vi "Memory.Pointer.Read.Safe.0D.I8.vi"(8 "error in (no error)":errorcluster, 10 "value in":i8, 11 "pointer in":refnum<class "Memory.Pointer.lvclass">) -> (0 "error out":errorcluster, 2 "value out":i8, 3 "pointer out":refnum<class "Memory.Pointer.lvclass">)   [LabVIEW 2016, in "Memory Manager.lvlib" / "Memory.Pointer.lvclass"]
doc: "Reads from the address specified by <b>pointer</b> into <b>value</b>.\n\n<b>Note:</b> This VI is <b>unsafe</b>.\n\nUnsafe means that it does not evaluate the size parameter of <b>pointer</b> to ensure that is inbounds of allocated memory before peforming a memory read/write. Reading/writing more data to a pointer than it has allocated can corrupt or crash LabVIEW. Only use this VI in scenarios where the <b>pointer</b> has been validated to be allocated to a correct size before calling this VI."
uses:
  Memory.Pointer.lvclass
  Memory.Pointer.lvclass/Memory.Pointer.ctl
  Accessors/Get Address.vi
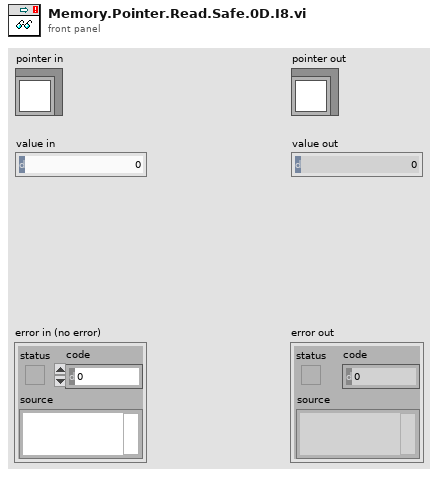
[diagram p1: front panel]
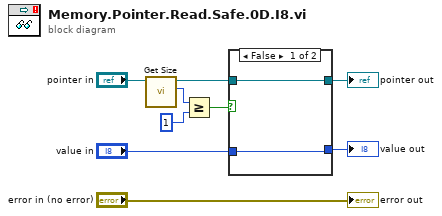
[diagram p0: block diagram]
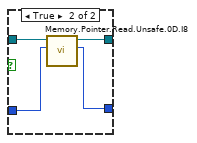
[diagram p2: hidden frame]
diagram:
  n1 = call "Get Size.vi"("Pointer in"="pointer in") -> ("size"=w8:u64, "Pointer out"=w5:refnum<class "Memory.Pointer.lvclass">)  [unwired: 8 in, 1 out]
  n2 = Greater Or Equal?(x=w8, y=u64 1) -> (x >= y?=w6:bool)
  n3 = case shown="False" w6 {
    tunnel: w5 -> [w11 w15]
    tunnel: [w11 w14] -> w4
    tunnel: "value in" -> [w10 w13]
    tunnel: [w10 w12] -> w2
    frame False {
    }
    frame True {
      n4 = call "Memory.Pointer.Read.Unsafe.0D.I8.vi"("value in"=w13, "pointer in"=w15) -> ("value out"=w12:i8, "pointer out"=w14:refnum<class "Memory.Pointer.lvclass">)  [unwired: 7 in, 1 out]
    }
  }
  "pointer out" <- w4
  "value out" <- w2
  "error out" <- "error in (no error)"
